vi "Decode Publish Package.vi"(7 "Type":variant, 8 "error in (no error)":errorcluster, 10 "PUBLISH in":refnum<class "PUBLISH.lvclass">, 11 "MQTT_Base in":refnum<class "MQTT_Base.lvclass">) -> (0 "error out":errorcluster, 1 "Payload":variant, 2 "Topic":string, 3 "MQTT_Base out":refnum<class "MQTT_Base.lvclass">)   [LabVIEW 2013, in "MQTT Base.lvlib" / "MQTT_Base.lvclass"]
uses:
  MQTT_Base.lvclass
  <vilib>/LabVIEW Open Source Project/MQTT Control Packets/Control Packets/PUBLISH/PUBLISH.lvclass
  MQTT_Base.lvclass/MQTT_Base.ctl
  <vilib>/LabVIEW Open Source Project/MQTT Control Packets/Control Packets/ControlPacket/ControlPacket.lvclass/ControlPacket.ctl
  <vilib>/LabVIEW Open Source Project/MQTT Control Packets/Control Packets/ControlPacket/ControlPacket.lvclass
  <vilib>/LabVIEW Open Source Project/Serializer/Serializer/Serializer.lvclass
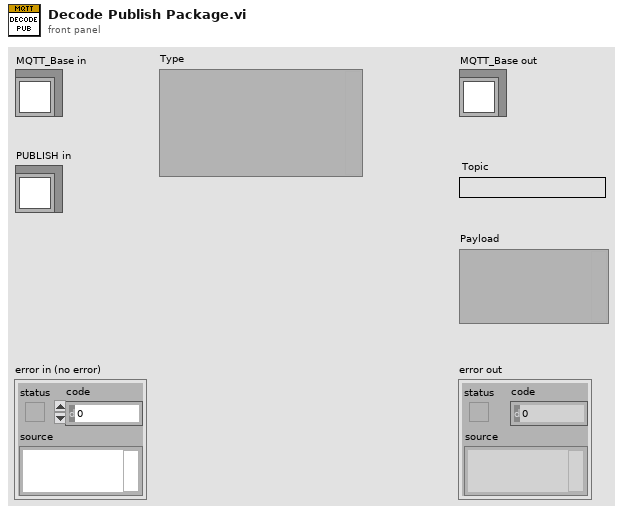
[diagram p1: front panel]
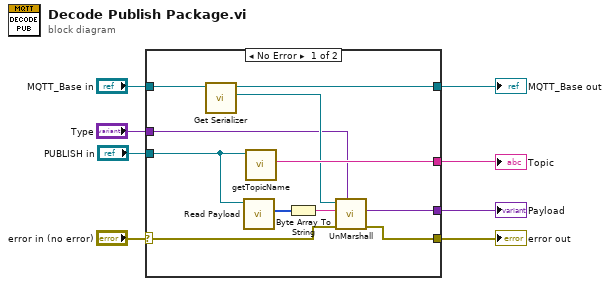
[diagram p0: block diagram]
diagram:
  n1 = case shown="No Error" "error in (no error)" {
    selector: "error in (no error)" -> [w13 w21]
    tunnel: [w14 w21] -> w7
    tunnel: [w11 w20] -> w5
    tunnel: "MQTT_Base in" -> [w12 w20]
    tunnel: "PUBLISH in" -> [w18 _]
    tunnel: [w19 _] -> w3
    tunnel: [w15 _] -> w2
    tunnel: "Type" -> [w9 _]
    frame No Error {
      n2 = call "Get Serializer.vi"("MQTT_Base"=w12) -> ("Serializer"=w10:refnum<class "Serializer.lvclass">, "MQTT_Base out"=w11:refnum<class "MQTT_Base.lvclass">)  [unwired: 8 in, 1 out]
      n3 = call <vilib>:"Read Payload.vi"("ControlPacket in"=w18) -> ("Payload"=w17:u8[])  [unwired: 9 in, 1 out]
      n4 = call <vilib>:"getTopicName.vi"("PUBLISH in"=w18) -> ("Topic"=w19:string)  [unwired: 8 in, 2 out]
      n5 = Byte Array To String(unsigned byte array=w17) -> (string=w16:string)
      n6 = call <vilib>:"UnMarshall.vi"("Type"=w9, "error in (no error)"=w13, "String"=w16, "Serializer in"=w10) -> ("error out"=w14:errorcluster, "Variant"=w15:variant)  [unwired: 5 in, 1 out]
    }
    frame Error {
    }
  }
  "error out" <- w7
  "MQTT_Base out" <- w5
  "Topic" <- w3
  "Payload" <- w2
